vi "Get XML Path.vi"(8 "error in (no error)":errorcluster, 11 "sbRIO-9651 in":refnum<class "sbRIO-9651.lvclass">) -> (0 "error out":errorcluster, 2 "XML Path":path, 3 "sbRIO-9651 out":refnum<class "sbRIO-9651.lvclass">)   [LabVIEW 2014, in "sbRIO-9651.lvclass"]
uses:
  sbRIO-9651.lvclass
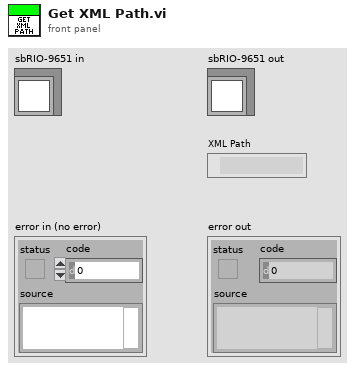
[diagram p1: front panel]
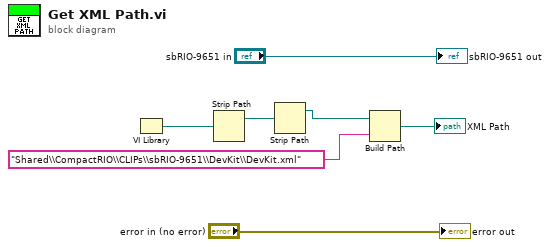
[diagram p0: block diagram]
diagram:
  n1 = VI Library() -> (path=w6:path)
  n2 = Strip Path(path=w6) -> (stripped path=w2:path)  [unwired: 1 out]
  n3 = Strip Path(path=w2) -> (stripped path=w1:path)  [unwired: 1 out]
  n4 = Build Path(base path=w1, name or relative path="Shared\\CompactRIO\\CLIPs\\sbRIO-9651\\DevKit\\DevKit.xml") -> (appended path=→"XML Path":path)
  "error out" <- "error in (no error)"
  "sbRIO-9651 out" <- "sbRIO-9651 in"
